vi "Keithly 2000 Global.vi"(7 "Mode (Read)":enum16{"Init", "Read DC Volts", "Close"}(ring)=enum."Read DC Volts", 8 "error in (no error)":errorcluster, 9 "# Samples (5)":i32=5, 10 "Timeout (1000 ms)":u32=1000, 11 "GPIB Reference":refnum<visa-resource-name>="GPIB0::0::INSTR") -> (0 "error out":errorcluster, 2 "Measurement":dbl)   [LabVIEW 2013]
uses:
  Keithly 2000 Support Files.llb/ke2000 Configure DC Volts.vi
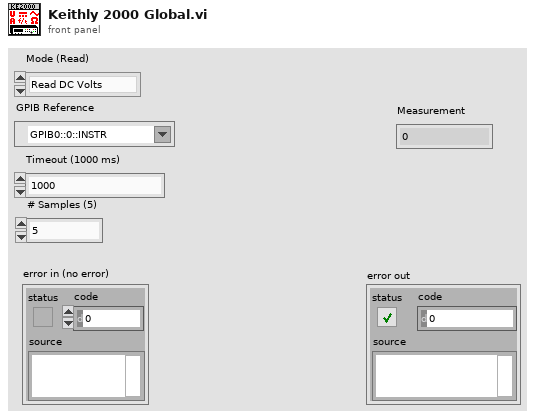
[diagram p1: front panel]
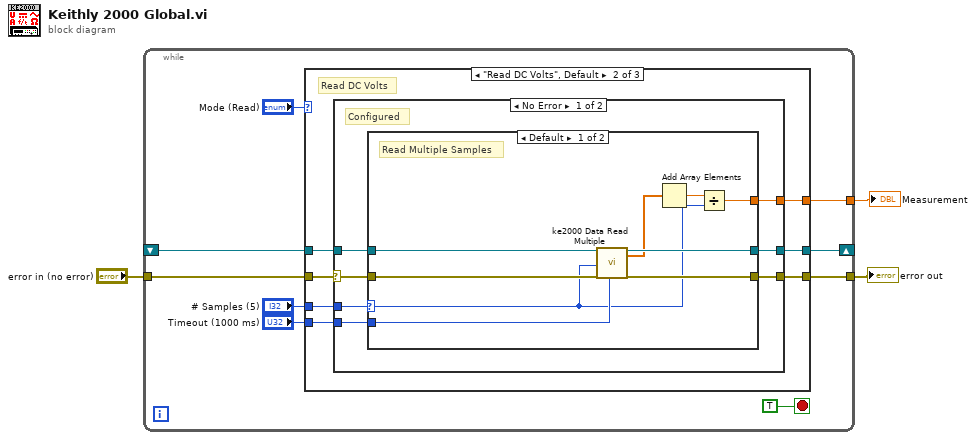
[diagram p0: block diagram]
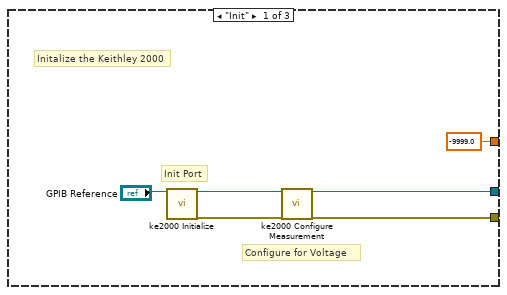
[diagram p2: hidden frame]
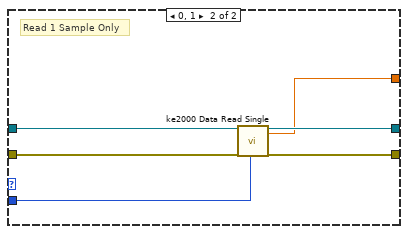
[diagram p3: hidden frame]
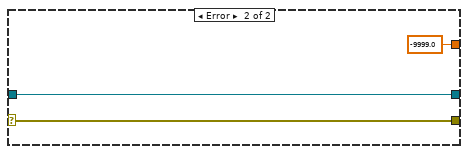
[diagram p4: hidden frame]
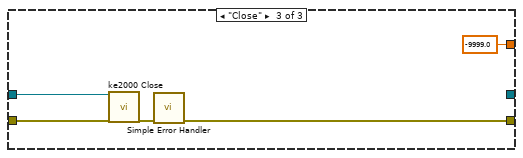
[diagram p5: hidden frame]
diagram:
  n1 = while {
    shift-right: [w10] -> _
    shift-left: _ -> [w8]
    tunnel: [w9] -> w3
    tunnel: "error in (no error)" -> [w4]
    tunnel: [w5] -> w1
    stop <- TRUE stop-if-true
    n2 = case shown="\"Read DC Volts\", Default" "Mode (Read)" {
      tunnel: [w16 w22 _] -> w10
      tunnel: [w13 w23 w52] -> w9
      tunnel: w8 -> [_ w24 w55]
      tunnel: "# Samples (5)" -> [_ w25 _]
      tunnel: "Timeout (1000 ms)" -> [_ w21 _]
      tunnel: [-9999.0 ("Measurement") w20 -9999.0 ("Measurement")] -> w5
      tunnel: w4 -> [_ w19 w54]
      frame "Init" {
        # "Init Port"
        # "Configure for Voltage"
        # "Initalize the Keithley 2000"
        n3 = call "ke2000 Initialize.vi"("VISA resource name"="GPIB Reference") -> ("VISA resource name out"=w17:refnum<visa-resource-name>, "error out"=w15:errorcluster)  [unwired: 17 in]
        n4 = call-poly "ke2000 Configure Measurement.vi"("VISA resource name"=w17, "error in (no error)"=w15) -> ("VISA resource name out"=w16:refnum<visa-resource-name>, "error out"=w13:errorcluster)  [unwired: 16 in]
      }
      frame "Read DC Volts", Default {
        # "Read DC Volts"
        n5 = case shown="No Error" w19 {
          selector: w19 -> [w26 w48]
          tunnel: w25 -> [w32 _]
          tunnel: w24 -> [w31 w49]
          tunnel: [w30 w48] -> w23
          tunnel: [w29 w49] -> w22
          tunnel: w21 -> [w28 _]
          tunnel: [w27 -9999.0 ("Measurement")] -> w20
          frame No Error {
            # "Configured"
            n6 = case shown="Default" w32 {
              selector: w32 -> [w34 _]
              tunnel: w31 -> [w41 w47]
              tunnel: w26 -> [w40 w46]
              tunnel: [w38 w45] -> w30
              tunnel: [w39 w44] -> w29
              tunnel: w28 -> [w37 w43]
              tunnel: [w33 w42] -> w27
              frame Default {
                # "Read Multiple Samples"
                n7 = call "ke2000 Data Read Multiple.vi"("VISA resource name"=w41, "Number of Readings (100)"=w34, "error in (no error)"=w40, "Timeout (25000 ms)"=w37) -> ("VISA resource name out"=w39:refnum<visa-resource-name>, "Data"=w36:dbl[], "error out"=w38:errorcluster)  [unwired: 11 in, 2 out]
                n8 = Add Array Elements(numeric array=w36) -> (sum=w35:dbl)
                n9 = Divide(x=w35, y=w34) -> (x/y=w33:dbl)
              }
              frame 0, 1 {
                # "Read 1 Sample Only"
                n10 = call "ke2000 Data Read Single.vi"("VISA resource name"=w47, "error in (no error)"=w46, "Timeout (25000 ms)"=w43) -> ("VISA resource name out"=w44:refnum<visa-resource-name>, "Measurement"=w42:dbl, "error out"=w45:errorcluster)  [unwired: 12 in, 2 out]
              }
            }
          }
          frame Error {
          }
        }
      }
      frame "Close" {
        n11 = call "ke2000 Close.vi"("VISA resource name"=w55, "error in (no error)"=w54) -> ("error out"=w53:errorcluster)  [unwired: 17 in]
        n12 = call <vilib>:"Simple Error Handler.vi"("error in (no error)"=w53) -> ("error out"=w52:errorcluster)  [unwired: 4 in, 4 out]
      }
    }
  }
  "error out" <- w3
  "Measurement" <- w1
